vi "AlliGator Check Fit Options.vi"(8 "error in (no error)":errorcluster, 9 "Modified Option":string="Use Data Information Laser Period", 10 "Use Data Information Period Refnum":refnum<vi>, 11 "Fit Options Refnum":refnum<vi>) -> (0 "error out":errorcluster, 3 "MLE Options Visible?":bool)   [LabVIEW 2021, in "AlliGator Settings.lvlib"]
doc: "Handles user-initiated parameter changes in the <B>Fit Options</B> panel."
uses:
  AlliGator Settings.lvlib
  Fits/IRF(X)PSED/Decay Fit Options v4.ctl
  Fits/Decay Convolution/Decay Model.ctl
  Fits/Residual Type.ctl
  Fits/IRF(X)PSED/Fit Weights Type v2.ctl
  Fits/Non-linear Fitting Method v2.ctl
  Fits/Fit Calculation Method.ctl
  Fits/Non-linear Fitting Algorithm.ctl
  Fits/Fit Settings.ctl
  Fits/Nonlinear Fit Method.ctl
  Fits/Ramp Type.ctl
  Fits/Fits.lvlib
panel:
  # "see the AlliGator License on the block diagram (Ctrl+E or Window:Show Block Diagram)"
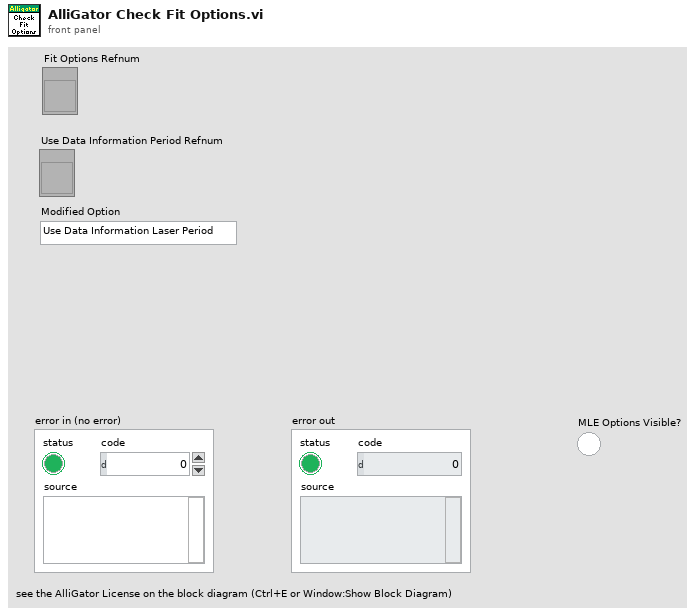
[diagram p1: front panel]
types:
  T1 = typedef "Fits.lvlib/Non-linear Fitting Method v2.ctl" = enum16{"Least Square", "Least Absolute Residual", "Bisquare", "MLE", "-", "Best of All"}
  T2 = typedef "Fits.lvlib/Decay Fit Options v4.ctl" = cluster{"Show Fit Residuals":bool, "Fit Model":T3, "Residual Type":T4, "Max Decay Percentile":dbl, "Min Decay Percentile":dbl, "Show Full Decay":bool, "Weights":T5, "Fitting Method":T1, "Compute Parameter Uncertainties":bool, "Periodic Boundaries":bool, "Model Calculation":T6, "Period":dbl[unit], "Termination Criteria":cluster{"Max Iterations":i32, "Max Function Calls":i32, "Max Time":dbl[unit], "Function Tolerance":dbl, "Parameter Tolerance":dbl, "Gradient Tolerance":dbl, "Min Lambda":dbl, "Max Lambda":dbl, "Initial Tick Count":u32}, "Offset Resolution":dbl[unit], "Use Local IRF":bool, "Fitting Algorithm":T7, "Show Confidence Interval ":bool, "Confidence Level":dbl}
  T3 = typedef "Fits.lvlib/Decay Model.ctl" = enum16{"1-Exponential", "2-Exponentials"}
  T4 = typedef "Fits.lvlib/Residual Type.ctl" = enum16{"Standard", "Normalized", "Reduced"}
  T5 = typedef "Fits.lvlib/Fit Weights Type v2.ctl" = enum16{"Unweighted", "1/Variance (Neyman)", "1/Variance (Pearson)", "Best of All"}
  T6 = typedef "Fits.lvlib/Fit Calculation Method.ctl" = enum16{"Simulation", "Convolution", "Integration"}
  T7 = typedef "Fits.lvlib/Non-linear Fitting Algorithm.ctl" = enum16{"Levenberg-Marquardt", "Trust-Region Dogleg"}
  T8 = typedef "Fits.lvlib/Fit Settings.ctl" = cluster{"Use Original Plot # Points":bool, "# Fit Plot Points":u32, "Fitting Method":T9, "Weighted Fit":T5, "Show All Fit Components":bool, "Axis Type":T10, "Show Fit Residuals":bool, "Residual Type":T4, "Fitting Algorithm":T7, "Show Confidence Interval":bool, "Confidence Level":dbl}
  T9 = typedef "Fits.lvlib/Nonlinear Fit Method.ctl" = enum16{"Least Square", "Least Absolute Residual", "Bisquare", "MLE"}
  T10 = typedef "Fits.lvlib/Ramp Type.ctl" = u16
  T11 = typedef "Fits.lvlib/D-Only Fixed Parameters.ctl" = cluster{"Fix D-only Peak Location":bool, "Peak Location":dbl, "Fix D-only Peak FWHM":bool, "Peak FWHM":dbl}
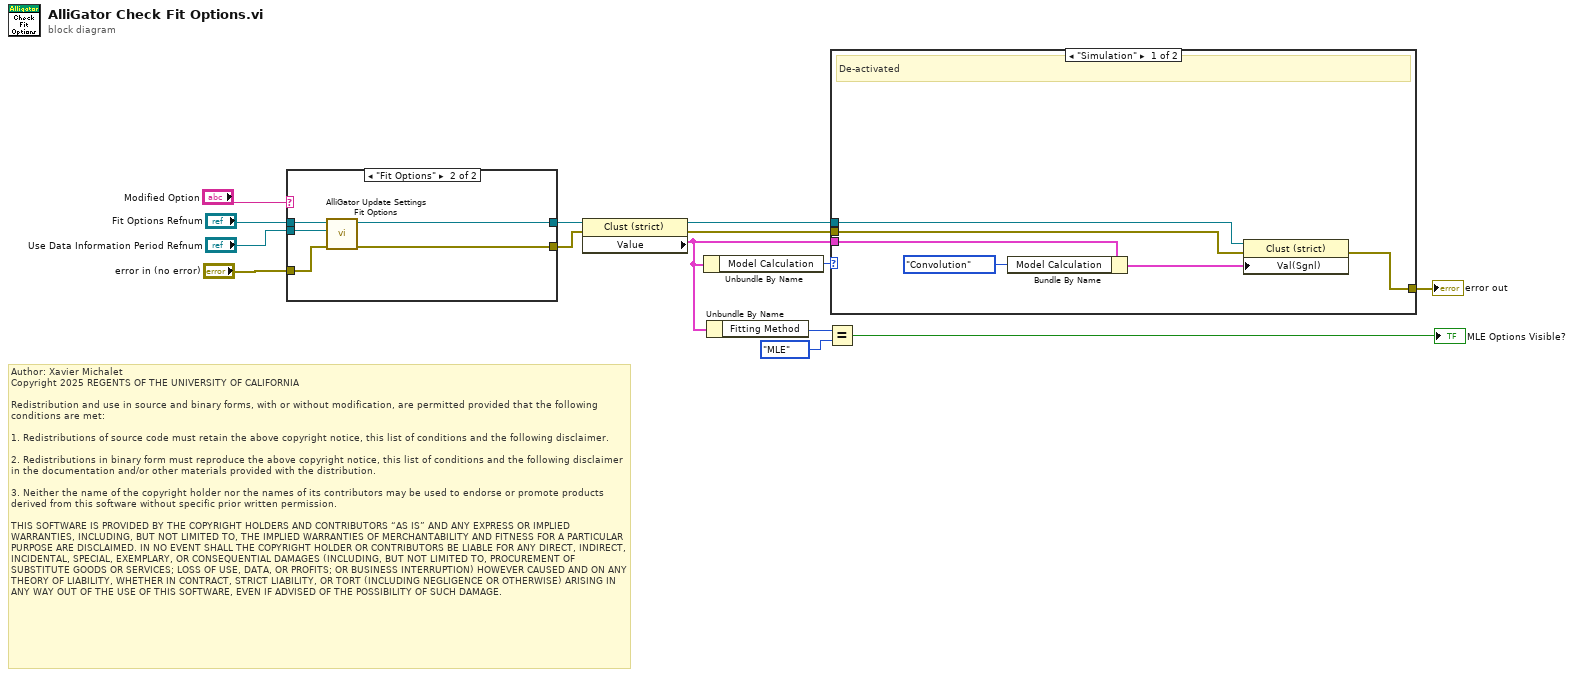
[diagram p0: block diagram]
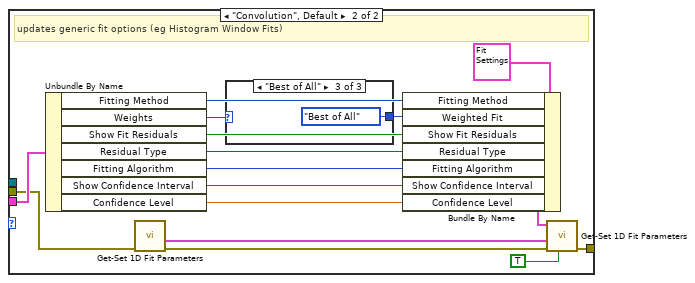
[diagram p2: hidden frame]
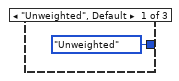
[diagram p3: hidden frame]
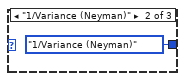
[diagram p4: hidden frame]
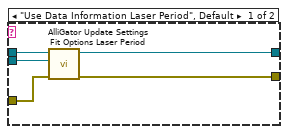
[diagram p5: hidden frame]
diagram:
  # "Author: Xavier Michalet\nCopyright 2025 REGENTS OF THE UNIVERSITY OF CALIFORNIA\n\nRedistribution and use in source and binary forms, with or without modification, are permitted provided that the following conditions are met:\n\n1. Redistributions of source code must retain the above copyright notice, this list of conditions and the following disclaimer.\n\n2. Redistributions in binary form must reproduce the above copyright notice, this list of conditions and the following disclaimer in the documentation and/or other materials provided with the distribution.\n\n3. Neither the name of the copyright holder nor the names of its contributors may be used to endorse or promote products derived from this software without specific prior written permission.\n\nTHIS SOFTWARE IS PROVIDED BY THE COPYRIGHT HOLDERS AND CONTRIBUTORS “AS IS” AND ANY EXPRESS OR IMPLIED WARRANTIES, INCLUDING, BUT NOT LIMITED TO, THE IMPLIED WARRANTIES OF MERCHANTABILITY AND FITNESS FOR A PARTICULAR PURPOSE ARE DISCLAIMED. IN NO EVENT SHALL THE COPYRIGHT HOLDER OR CONTRIBUTORS BE LIABLE FOR ANY DIRECT, INDIRECT, INCIDENTAL, SPECIAL, EXEMPLARY, OR CONSEQUENTIAL DAMAGES (INCLUDING, BUT NOT LIMITED TO, PROCUREMENT OF SUBSTITUTE GOODS OR SERVICES; LOSS OF USE, DATA, OR PROFITS; OR BUSINESS INTERRUPTION) HOWEVER CAUSED AND ON ANY THEORY OF LIABILITY, WHETHER IN CONTRACT, STRICT LIABILITY, OR TORT (INCLUDING NEGLIGENCE OR OTHERWISE) ARISING IN ANY WAY OUT OF THE USE OF THIS SOFTWARE, EVEN IF ADVISED OF THE POSSIBILITY OF SUCH DAMAGE."
  n1 = case shown="\"Fit Options\"" "Modified Option" {
    tunnel: [w19 w24] -> w12
    tunnel: "error in (no error)" -> [w18 w23]
    tunnel: [w17 w22] -> w5
    tunnel: "Fit Options Refnum" -> [w16 w21]
    tunnel: "Use Data Information Period Refnum" -> [w15 w20]
    frame "Use Data Information Laser Period", Default {
      n2 = call "AlliGator Update Settings Fit Options Laser Period.vi"("error in (no error)"=w18, "Use Data Information Laser Period Refnum"=w15, "Fit Options Refnum"=w16) -> ("error out"=w17:errorcluster, "Fit Options Refnum"=w19:refnum<vi>)  [unwired: 7 in]
    }
    frame "Fit Options" {
      n3 = call "AlliGator Update Settings Fit Options.vi"("error in (no error)"=w23, "Use Data Information Laser Period Refnum"=w20, "Fit Options Refnum"=w21) -> ("error out"=w22:errorcluster, "Fit Options Refnum"=w24:refnum<vi>)  [unwired: 7 in]
    }
  }
  n4 = property class="Clust (strict)"(reference=w12, error in=w5) -> (reference out=w10:refnum<vi>, error out=w4:errorcluster, "Value"=w6:T2)
  n5 = Unbundle By Name(w6) -> ("Model Calculation"=w14:T6)
  n6 = Unbundle By Name(w6) -> ("Fitting Method"=w3:T1)
  n7 = Equal?(x=w3, y=Non-linear_Fitting_Method_v2."MLE") -> (x = y?=→"MLE Options Visible?":bool)
  n8 = case shown="\"Simulation\"" w14 {
    tunnel: w6 -> [w30 w44]
    tunnel: w10 -> [w28 _]
    tunnel: [w26 w46] -> w13
    tunnel: w4 -> [w25 w35]
    frame "Simulation" {
      # "De-activated"
      n9 = Bundle By Name(cluster=w30, "Model Calculation"=Fit_Calculation_Method."Convolution" ("Method")) -> (w27:T2)
      n10 = property class="Clust (strict)"(reference=w28, error in=w25, "Val(Sgnl)"=w27) -> (error out=w26:errorcluster)  [unwired: 1 out]
    }
    frame "Convolution", Default {
      # "updates generic fit options (eg Histogram Window Fits)"
      n11 = Unbundle By Name(w44) -> ("Fitting Method"=w39:T1, "Weights"=w32:T5, "Show Fit Residuals"=w38:bool, "Residual Type"=w37:T4, "Fitting Algorithm"=w36:T7, "Show Confidence Interval"=w34:bool, "Confidence Level"=w33:dbl)
      n12 = call "Get-Set 1D Fit Parameters.vi"("Error In"=w35) -> ("Error Out"=w43:errorcluster, "Fixed Parameters"=w42:T11)  [unwired: 7 in, 2 out]
      n13 = case shown="\"Best of All\"" w32 {
        tunnel: [Fit_Weights_Type_v2."Unweighted" ("Weighted Fit") Fit_Weights_Type_v2."1/Variance (Neyman)" ("Weighted Fit") Fit_Weights_Type_v2."Best of All" ("Weighted Fit")] -> w31
        frame "Unweighted", Default {
        }
        frame "1/Variance (Neyman)" {
        }
        frame "Best of All" {
        }
      }
      n14 = Bundle By Name(cluster=T8 {"Use Original Plot # Points"=FALSE, "# Fit Plot Points"=1000, "Fitting Method"=enum."Least Square", "Weighted Fit"=enum."1/Variance (Neyman)", "Show All Fit Components"=FALSE, "Axis Type"=0, "Show Fit Residuals"=FALSE, "Residual Type"=enum."Standard", "Fitting Algorithm"=enum."Levenberg-Marquardt", "Show Confidence Interval"=TRUE, "Confidence Level"=95.0} ("Fit Settings"), "Fitting Method"=w39, "Weighted Fit"=w31, "Show Fit Residuals"=w38, "Residual Type"=w37, "Fitting Algorithm"=w36, "Show Confidence Interval"=w34, "Confidence Level"=w33) -> (w40:T8)
      n15 = call "Get-Set 1D Fit Parameters.vi"("Get(F)/Set"=TRUE, "Error In"=w43, "Fixed Parameters"=w42, "Fit Settings"=w40) -> ("Error Out"=w46:errorcluster)  [unwired: 4 in, 3 out]
    }
  }
  "error out" <- w13
